vi "MQTT_SUBS.vi"(8 "error in (no error)":errorcluster, 9 "TOPIC":string, 10 "IP":string, 11 "VISA resource name":refnum<visa-resource-name>) -> (0 "error out":errorcluster, 1 "Lectura MQTT":string, 3 "VISA resource name out":refnum<visa-resource-name>)   [LabVIEW 2025]
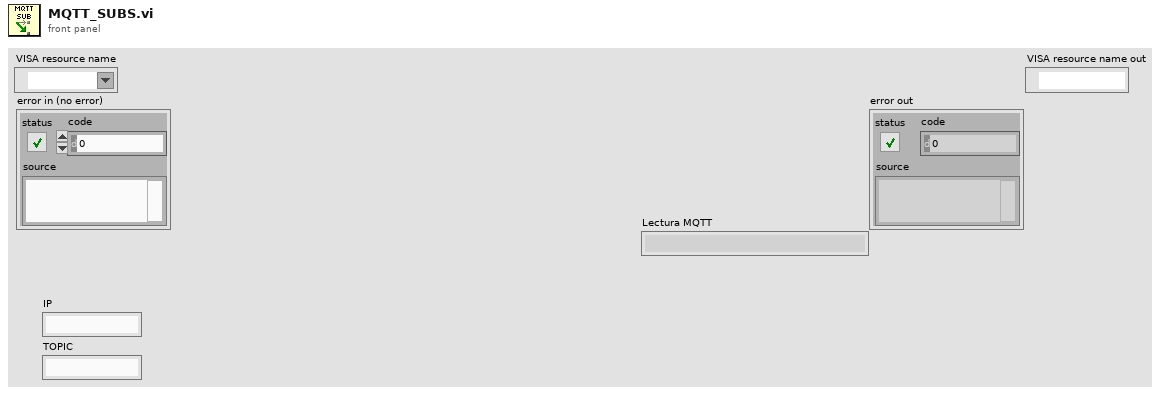
[diagram p1: front panel]
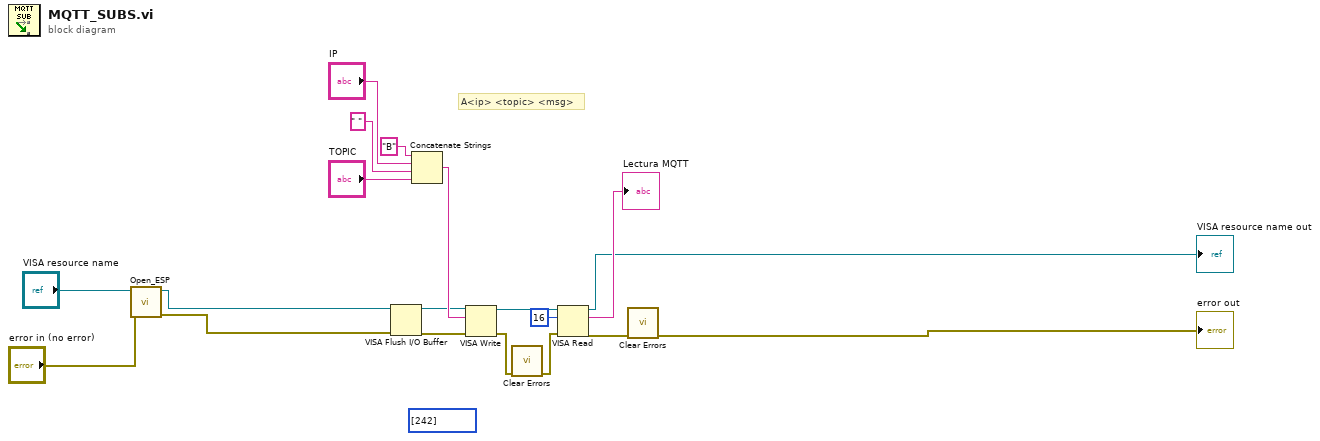
[diagram p0: block diagram]
diagram:
  (unwired) u8[] [242]
  # "A<ip> <topic> <msg>"
  n1 = call "Open_ESP.vi"("error in (no error)"="error in (no error)", "VISA resource name"="VISA resource name") -> ("error out"=w18:errorcluster, "VISA resource name out"=w19:refnum<visa-resource-name>)  [unwired: 8 in]
  n2 = VISA Flush I/O Buffer(VISA resource name=w19, error in (no error)=w18) -> (VISA resource name out=w9:refnum<visa-resource-name>, error out=w8:errorcluster)  [unwired: 1 in]
  n3 = Concatenate Strings("B", "IP", " " ("string"), "TOPIC") -> (w12:string)
  n4 = VISA Write(VISA resource name=w9, write buffer=w12, error in (no error)=w8) -> (VISA resource name out=w16:refnum<visa-resource-name>, error out=w6:errorcluster)  [unwired: 1 out]
  n5 = call <vilib>:"Clear Errors.vi"("error in (no error)"=w6) -> ("error out"=w5:errorcluster)  [unwired: 5 in, 1 out]
  n6 = VISA Read(VISA resource name=w16, byte count=u32 16, error in (no error)=w5) -> (VISA resource name out=→"VISA resource name out":refnum<visa-resource-name>, read buffer=→"Lectura MQTT":string, error out=w4:errorcluster)  [unwired: 1 out]
  n7 = call <vilib>:"Clear Errors.vi"("error in (no error)"=w4) -> ("error out"=→"error out":errorcluster)  [unwired: 5 in, 1 out]
